vi "iV programa 2_2.vi"() -> ()   [LabVIEW 2020]
panel:
  out "max index(es)":i32
  out "min value":dbl
  out "max value":dbl
  out "C°     F°":dbl[][](array[numeric])
  out "N, C°":cluster{i32[], dbl[]}(graph)
  # "2.2. Genere un instrumento virtual que simule la adquisición de temperatura. Considere lo siguiente:\n• Genere 100 datos aleatorias dentro de un rango de 0 a 45.\n• Grafique los datos obtenidos.\n• Almacene los datos en un arreglo donde la primera columna deberá contener los datos originales, la segunda columna los datos representados en grados Fahrenheit.\n• La tercera columna los datos a la salida de un filtro EMA.\n• Un indicador que muestre el número máximo.\n• Otro indicador que muestre el valor mínimo."
  # "100 muestras de temperatura graficadas en escala de C°"
  # "C°      F°      F° EMA"
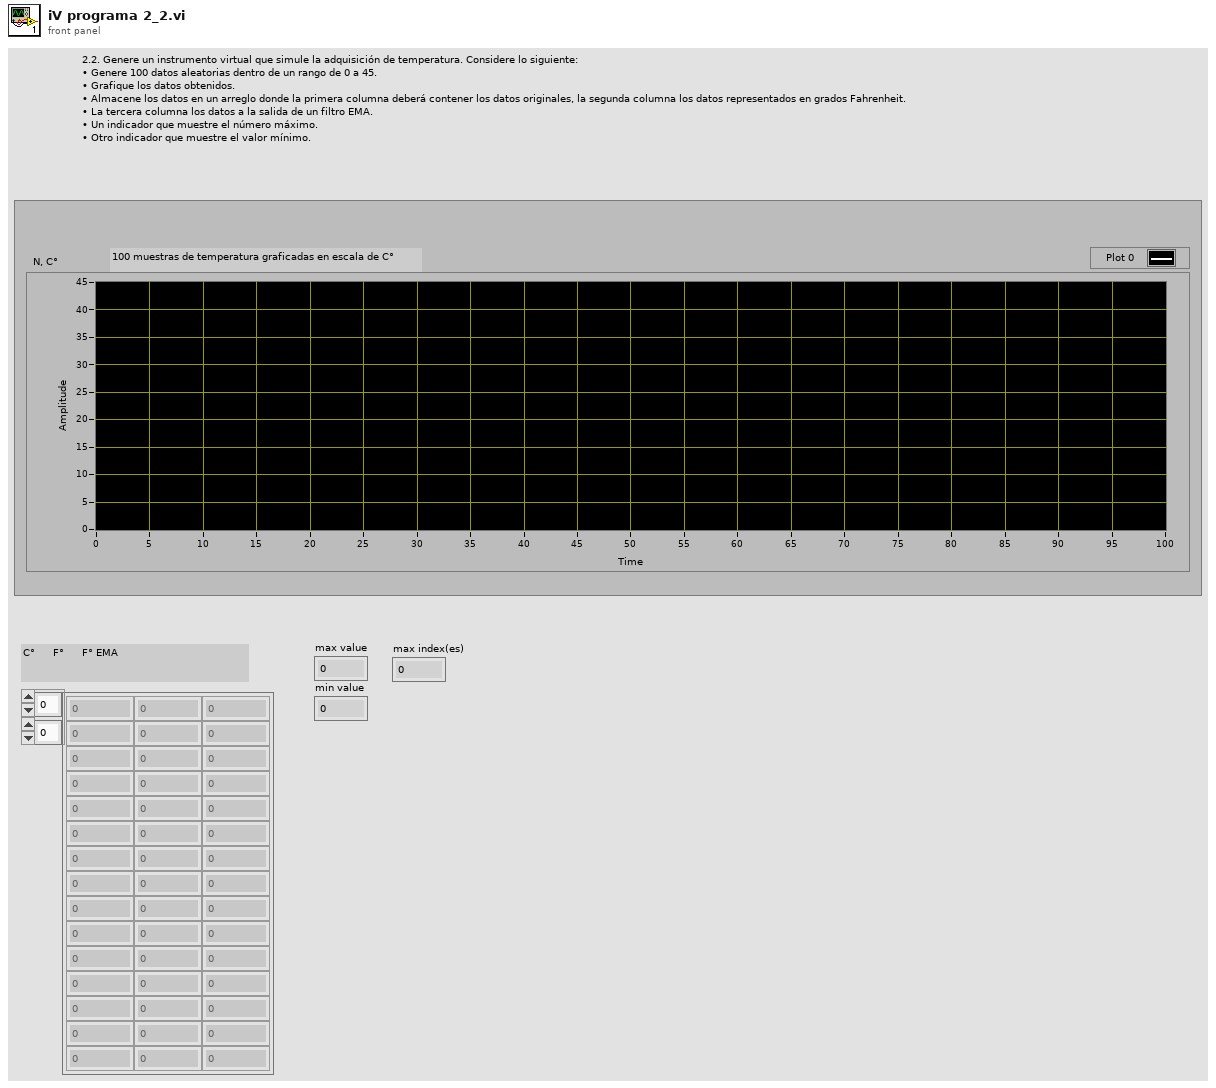
[diagram p1: front panel]
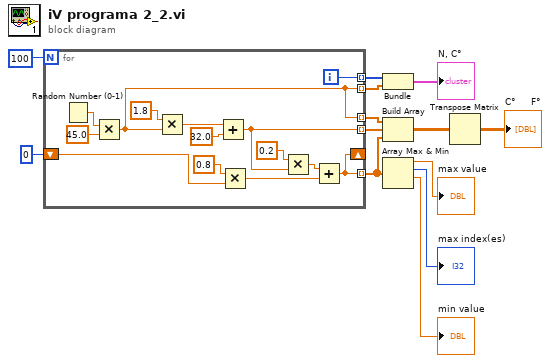
[diagram p0: block diagram]
diagram:
  n1 = for {
    N: 100 -> [_]
    tunnel: [w21] -> w10 mode=indexing
    tunnel: [w25] -> w11 mode=indexing
    tunnel: [w20] -> w8 mode=indexing
    tunnel: [w21] -> w9 mode=indexing
    shift-right: [w14] -> _
    shift-left: 0 -> [w16]
    tunnel: [w14] -> w2 mode=indexing
    i -> [w25]
    n2 = Random Number (0-1)() -> (number: 0 to 1=w27:dbl)
    n3 = Multiply(x=w27, y=45.0) -> (x*y=w21:dbl)
    n4 = Multiply(x=1.8, y=w21) -> (x*y=w23:dbl)
    n5 = Add(x=w23, y=32.0) -> (x+y=w20:dbl)
    n6 = Multiply(x=0.8, y=w16) -> (x*y=w15:dbl)
    n7 = Multiply(x=0.2, y=w20) -> (x*y=w18:dbl)
    n8 = Add(x=w18, y=w15) -> (x+y=w14:dbl)
  }
  n9 = Bundle(w11, w10) -> (→"N, C°":cluster{i32[], dbl[]})  [unwired: 1 in]
  n10 = Build Array(w9, w8, w2) -> (w6:dbl[][])
  n11 = Array Max & Min(array=w2) -> (max value=→"max value":dbl, max index (indices)=→"max index(es)":i32, min value=→"min value":dbl)  [unwired: 1 out]
  n12 = Transpose Matrix(1:w6) -> (0:→"C°     F°":dbl[][])
